vi "Terminate Condition Extract Time Condition C.vi"(7 "Conditions":T8, 8 "error in":errorcluster, 11 "PLC Data In":T1 {"PLC Data - LDO"."Timing"."Absolute Time" format="%<%H:%M:%S%3u>t"; "PLC Data - LDO"."Timing"."Display Time" format="%#.20f"; "PLC Data - LDO"."Timing"."Test Time Ref" format="%#.20f"; "PLC Data - LDO"."Timing"."Precondition Time Ref" format="%#.20f"; "PLC Data - LDO"."Timing"."First Call Time Ref" format="%#.20f"; "PLC Data - FVIR"."Timing"."Absolute Time" format="%<%H:%M:%S%3u>t"; "PLC Data - FVIR"."Timing"."Display Time" format="%#.20f"; "PLC Data - FVIR"."Timing"."Test Time Ref" format="%#.20f"; "PLC Data - FVIR"."Timing"."Precondition Time Ref" format="%#.20f"; "PLC Data - FVIR"."Timing"."First Call Time Ref" format="%#.20f"}) -> (0 "error out":errorcluster, 3 "PLC Data Out":T1 {"PLC Data - LDO"."Timing"."Absolute Time" format="%<%H:%M:%S%3u>t"; "PLC Data - LDO"."Timing"."Display Time" format="%#.20f"; "PLC Data - LDO"."Timing"."Test Time Ref" format="%#.20f"; "PLC Data - LDO"."Timing"."Precondition Time Ref" format="%#.20f"; "PLC Data - LDO"."Timing"."First Call Time Ref" format="%#.20f"; "PLC Data - FVIR"."Timing"."Absolute Time" format="%<%H:%M:%S%3u>t"; "PLC Data - FVIR"."Timing"."Display Time" format="%#.20f"; "PLC Data - FVIR"."Timing"."Test Time Ref" format="%#.20f"; "PLC Data - FVIR"."Timing"."Precondition Time Ref" format="%#.20f"; "PLC Data - FVIR"."Timing"."First Call Time Ref" format="%#.20f"})   [LabVIEW 2023]
uses:
  Terminate Condition ENUM.ctl
  Modbus/Modbus PLC Data All.ctl
  Modbus/Modbus FVIR Control.ctl
  Modbus/Modbus Timing.ctl
  <vilib>/Utility/miscctls.llb/LVDateTimeRec.ctl
  Modbus/Modbus LDO Control.ctl
  WritingDataFile/Data to Save.ctl
  Terminate Conditions Cluster.ctl
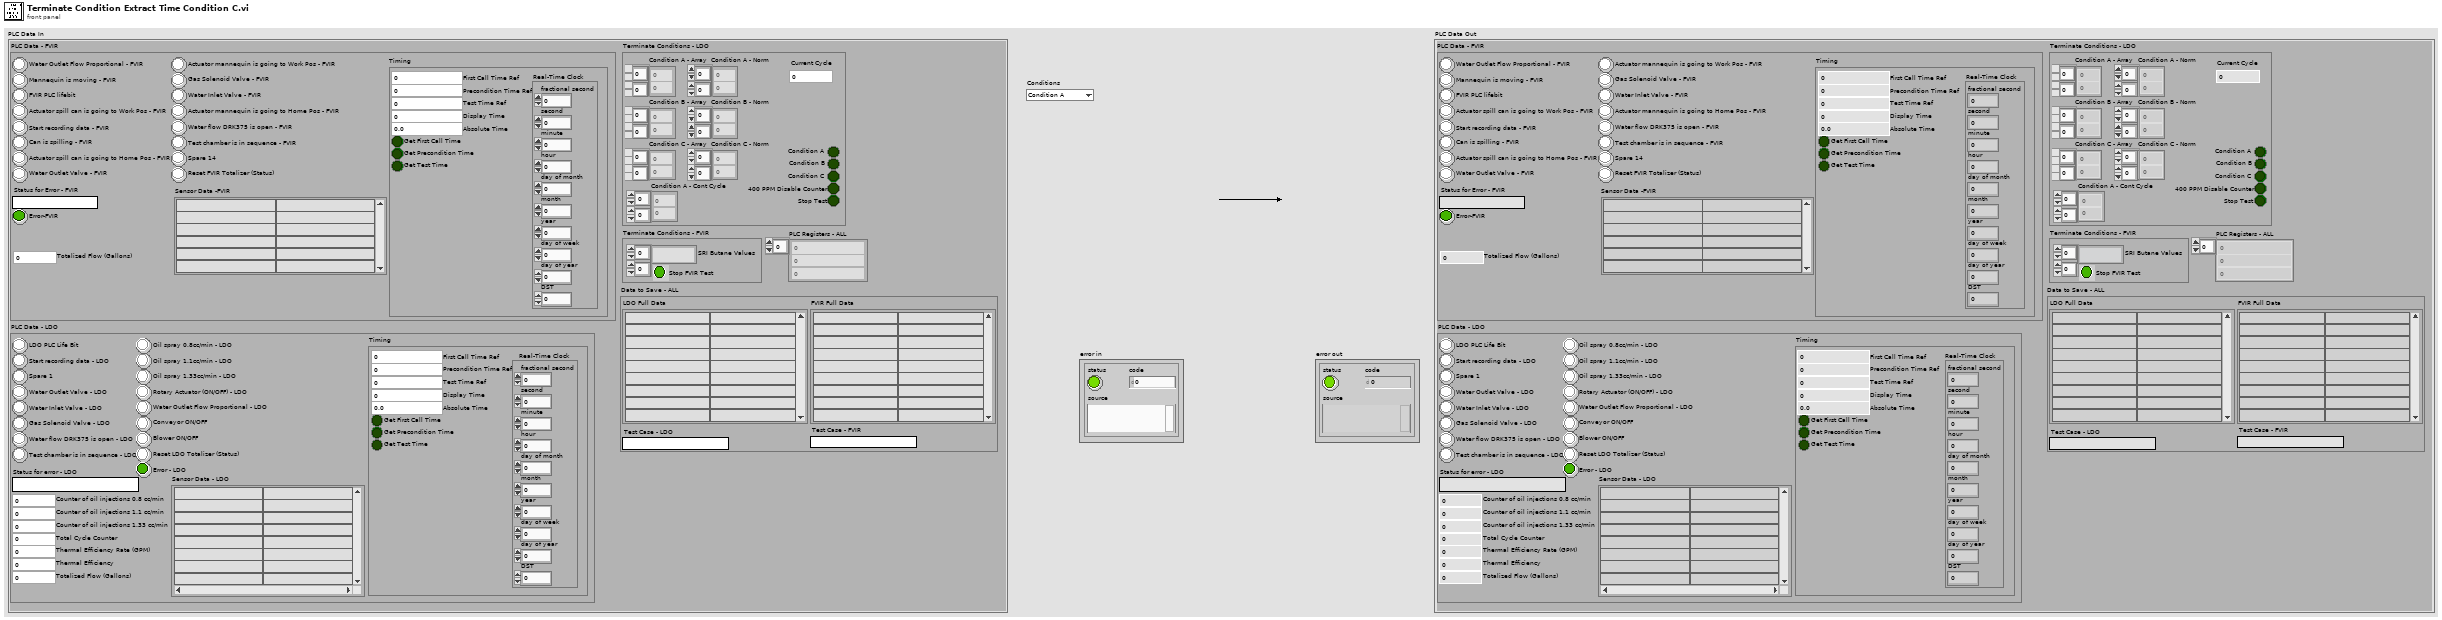
[diagram p1: front panel]
types:
  T1 = typedef "Modbus PLC Data All.ctl" = cluster{"PLC Data - FVIR":T2, "PLC Data - LDO":T5, "PLC Registers - ALL":i16[], "Data to Save - ALL":T6, "Terminate Conditions - LDO":T7, "Terminate Conditions - FVIR":cluster{"SRI Butane Values":string[][], "Stop FVIR Test":bool}}
  T2 = typedef "Modbus FVIR Control.ctl" = cluster{"Reset FVIR Totalizer (Status)":bool, "Spare 14":bool, "Actuator mannequin is going to Work Pos - FVIR":bool, "Actuator mannequin is going to Home Pos - FVIR":bool, "Test chamber is in sequence - FVIR ":bool, "Water flow DRK375 is open - FVIR":bool, "Gas Solenoid Valve - FVIR":bool, "Water Inlet Valve - FVIR":bool, "Water Outlet Flow Proportional - FVIR":bool, "Start recording data - FVIR":bool, "Actuator spill can is going to Work Pos - FVIR":bool, "Actuator spill can is going to Home Pos - FVIR":bool, "Water Outlet Valve - FVIR":bool, "Can is spilling - FVIR":bool, "Mannequin is moving - FVIR":bool, "FVIR PLC lifebit":bool, "Status for Error - FVIR":string, "Error-FVIR":bool, "Sensor Data -FVIR":string[][], "Totalized Flow (Gallons)":dbl, "Timing":T3}
  T3 = typedef "Modbus Timing.ctl" = cluster{"First Call Time Ref":dbl, "Precondition Time Ref":dbl, "Test Time Ref":dbl, "Get First Call Time":bool, "Get Precondition Time":bool, "Get Test Time":bool, "Display Time":dbl, "Real-Time Clock":T4, "Absolute Time":dbl}
  T4 = typedef "LVDateTimeRec.ctl" = cluster{"fractional second":dbl, "second":i32, "minute":i32, "hour":i32, "day of month":i32, "month":i32, "year":i32, "day of week":i32, "day of year":i32, "DST":i32}
  T5 = typedef "Modbus LDO Control.ctl" = cluster{"LDO PLC Life Bit":bool, "Start recording data - LDO":bool, "Spare 1":bool, "Water Outlet Valve - LDO":bool, "Water Inlet Valve - LDO":bool, "Gas Solenoid Valve - LDO":bool, "Water flow DRK375 is open - LDO":bool, "Test chamber is in sequence - LDO":bool, "Oil spray 0.8cc/min - LDO":bool, "Oil spray 1.1cc/min - LDO":bool, "Oil spray 1.33cc/min - LDO":bool, "Rotary Actuator (ON/OFF) - LDO":bool, "Water Outlet Flow Proportional - LDO":bool, "Conveyor ON/OFF":bool, "Blower ON/OFF":bool, "Reset LDO Totalizer (Status)":bool, "Status for error - LDO":string, "Error - LDO":bool, "Sensor Data - LDO":string[][], "Thermal Efficiency Rate (GPM)":dbl, "Thermal Efficiency":dbl, "Totalized Flow (Gallons)":dbl, "Counter of oil injections 1.33 cc/min":u16, "Total Cycle Counter":u16, "Counter of oil injections 1.1 cc/min":u16, "Counter of oil injections 0.8 cc/min":u16, "Timing":T3}
  T6 = typedef "Data to Save.ctl" = cluster{"LDO Full Data":string[][], "FVIR Full Data":string[][], "Test Case - FVIR":string, "Test Case - LDO":string}
  T7 = typedef "Terminate Conditions Cluster.ctl" = cluster{"Condition B - Array":dbl[][], "Current Cycle":u16, "Condition C - Array":dbl[][], "Condition A - Array":dbl[][], "400 PPM Disable Counter":bool, "Condition A - Norm":dbl[][], "Condition B - Norm":dbl[][], "Condition C - Norm":dbl[][], "Condition A":bool, "Condition B":bool, "Condition C":bool, "Condition A - Cont Cycle":dbl[][], "Stop Test":bool}
  T8 = typedef "Terminate Condition ENUM.ctl" = enum16{"Condition A", "Condition B", "Condition C"}
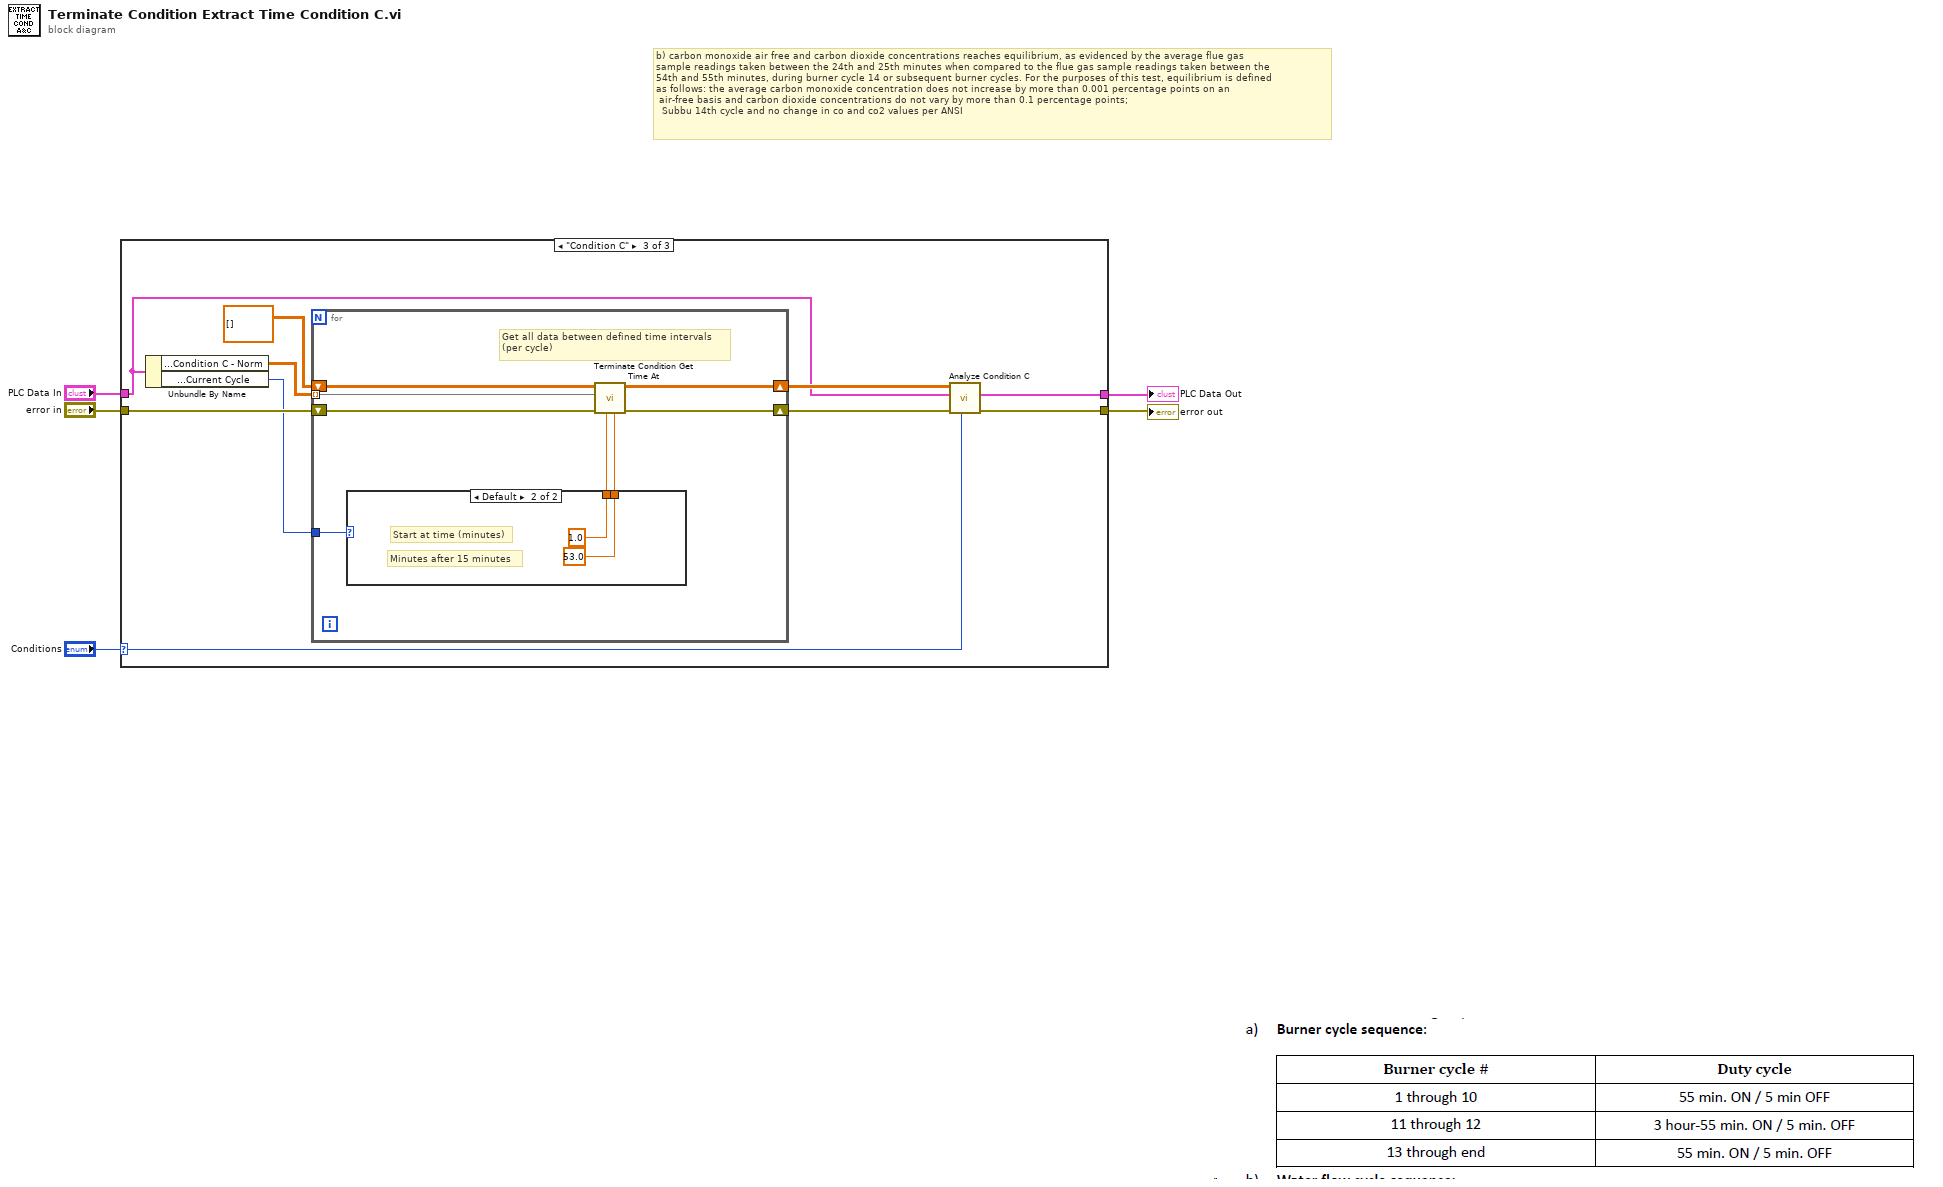
[diagram p0: block diagram]
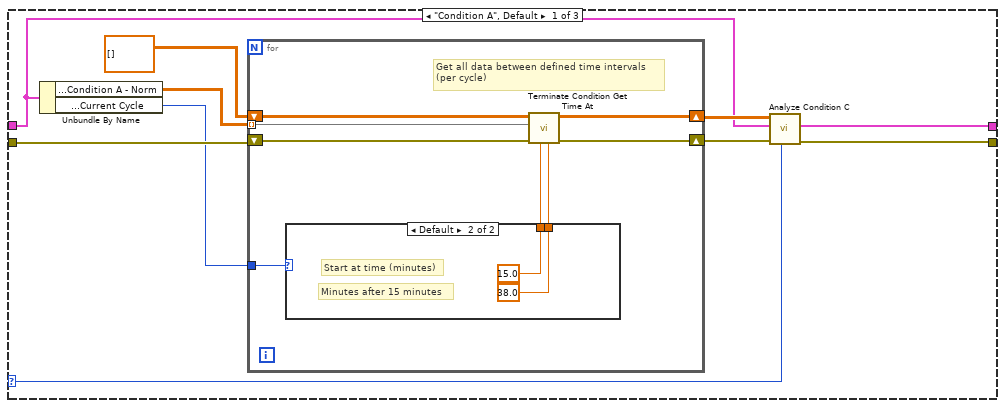
[diagram p2: hidden frame]
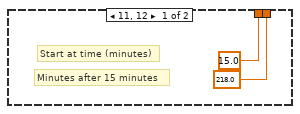
[diagram p3: hidden frame]
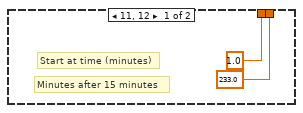
[diagram p5: hidden frame]
diagram:
  # "b) carbon monoxide air free and carbon dioxide concentrations reaches equilibrium, as evidenced by the average flue gas\nsample readings taken between the 24th and 25th minutes when compared to the flue gas sample readings taken between the\n54th and 55th minutes, during burner cycle 14 or subsequent burner cycles. For the purposes of this test, equilibrium is defined\nas follows: the average carbon monoxide concentration does not increase by more than 0.001 percentage points on an\n air-free basis and carbon dioxide concentrations do not vary by more than 0.1 percentage points;\n  Subbu 14th cycle and no change in co and co2 values per ANSI"
  n1 = case shown="\"Condition C\"" "Conditions" {
    selector: "Conditions" -> [w6 _ w30]
    tunnel: "PLC Data In" -> [w7 w28 w33]
    tunnel: "error in" -> [w13 w29 w37]
    tunnel: [w11 w29 w34] -> w1
    tunnel: [w8 w28 w32] -> w2
    frame "Condition A", Default {
      n2 = Unbundle By Name(w7) -> ("Terminate Conditions - LDO.Condition A - Norm"=w14:dbl[][], "Terminate Conditions - LDO.Current Cycle"=w9:u16)
      n3 = for {
        tunnel: w14 -> [w21] mode=indexing
        shift-right: [w22] -> w10
        shift-left: dbl[][] [] -> [w23]
        shift-right: [w19] -> w12
        shift-left: w13 -> [w20]
        tunnel: w9 -> [w16]
        # "Get all data between defined time intervals \n(per cycle)"
        n4 = case shown="Default" w16 {
          tunnel: [15.0 ("Get Time At (Min)") 15.0 ("Get Time At (Min)")] -> w18
          tunnel: [218.0 ("Minute Adder") 38.0 ("Minute Adder")] -> w17
          frame 11, 12 {
            # "Minutes after 15 minutes"
            # "Start at time (minutes)"
          }
          frame Default {
            # "Minutes after 15 minutes"
            # "Start at time (minutes)"
          }
        }
        n5 = call "Terminate Condition Get Time At.vi"("Minute Adder"=w17, "Get Time At (Min)"=w18, "error in"=w20, "Normalized Timer Array in"=w21, "Array in"=w23) -> ("error out"=w19:errorcluster, "Array out"=w22:dbl[][])  [unwired: 5 in]
      }
      n6 = call "Analyze Condition C.vi"("Conditions"=w6, "error in"=w12, "PLC Data In"=w7, "Condition Array"=w10) -> ("error out"=w11:errorcluster, "PLC Data Out"=w8:T1)  [unwired: 6 in]
    }
    frame "Condition B" {
    }
    frame "Condition C" {
      n7 = Unbundle By Name(w33) -> ("Terminate Conditions - LDO.Condition C - Norm"=w38:dbl[][], "Terminate Conditions - LDO.Current Cycle"=w31:u16)
      n8 = for {
        tunnel: w38 -> [w44] mode=indexing
        shift-right: [w46] -> w36
        shift-left: dbl[][] [] -> [w47]
        shift-right: [w41] -> w35
        shift-left: w37 -> [w42]
        tunnel: w31 -> [w40]
        # "Get all data between defined time intervals \n(per cycle)"
        n9 = case shown="Default" w40 {
          tunnel: [1.0 ("Get Time At (Min)") 1.0 ("Get Time At (Min)")] -> w45
          tunnel: [233.0 ("Minute Adder") 53.0 ("Minute Adder")] -> w43
          frame 11, 12 {
            # "Minutes after 15 minutes"
            # "Start at time (minutes)"
          }
          frame Default {
            # "Minutes after 15 minutes"
            # "Start at time (minutes)"
          }
        }
        n10 = call "Terminate Condition Get Time At.vi"("Minute Adder"=w43, "Get Time At (Min)"=w45, "error in"=w42, "Normalized Timer Array in"=w44, "Array in"=w47) -> ("error out"=w41:errorcluster, "Array out"=w46:dbl[][])  [unwired: 5 in]
      }
      n11 = call "Analyze Condition C.vi"("Conditions"=w30, "error in"=w35, "PLC Data In"=w33, "Condition Array"=w36) -> ("error out"=w34:errorcluster, "PLC Data Out"=w32:T1)  [unwired: 6 in]
    }
  }
  "error out" <- w1
  "PLC Data Out" <- w2
